vi "Test Fails.vi"(11 "Test Case In":refnum<class "Example Test.lvclass">) -> (0 "error out":errorcluster, 3 "Test Case Out":refnum<class "Example Test.lvclass">)   [LabVIEW 2021, in "Example Test.lvclass"]
uses:
  Example Test.lvclass
  C:/Program Files (x86)/National Instruments/LabVIEW 2026/vi.lib/Astemes/LUnit/Test Case.lvclass
  <vilib>/Astemes/LUnit/Test Case.lvclass/Test Case.ctl
  Example Test.lvclass/Example Test.ctl
  51246cad-6428-43d3-a87d-9ed933ddf7be.vi
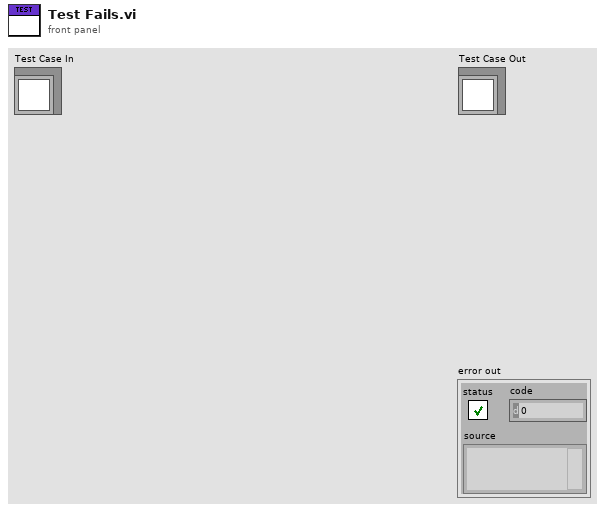
[diagram p1: front panel]
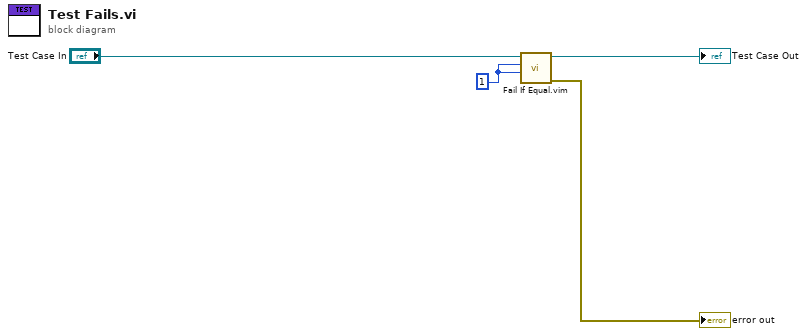
[diagram p0: block diagram]
diagram:
  w1 = 1
  n1 = call "Fail If Equal.vim"("Actual"=w1, "Unexpected"=w1, "LUnit Test Case In"="Test Case In") -> ("error out"=→"error out":errorcluster, "LUnit Test Case Out"=→"Test Case Out":refnum<class "Example Test.lvclass">)  [unwired: 7 in]
